vi "ASC-FlowControl.vi"() -> ()   [LabVIEW 2009]
uses:
  <vilib>/Utility/error.llb/DialogType.ctl
  Time_globals.vi
  Instance           4 19Saved   Wetlow_v1.2 .vi
panel:
  out "Flush":bool
  out "Progress":string
  in  "Fugacity table":dbl[](array[numeric])
  in  "Temperature table":dbl[](array[numeric])
  out "Fugacity":cluster{"Array":dbl[], "Array 2":dbl[]}[](graph)=[{"Array"=[17.44743958824043, 17.44743958824043], "Array 2"=[-15.0, -90.0]}, {"Array"=[14.85552997103172, 14.85552997103172], "Array 2"=[-15.0, -90.0]}, {"Array"=[12.93410075664489, 12.93410075664489], "Array 2"=[-15.0, -90.0]}, {"Array"=[11.45278589016778, 11.45278589016778], "Array 2"=[-15.0, -90.0]}, {"Array"=[10.27590813338129, 10.27590813338129], "Array 2"=[-15.0, -90.0]}, {"Array"=[9.318361831989936, 9.318361831989936], "Array 2"=[-15.0, -90.0]}, {"Array"=[21.13, 21.13], "Array 2"=[-15.0, -90.0]}, {"Array"=[26.8, 26.8], "Array 2"=[-15.0, -90.0]}, {"Array"=[33.65, 33.65], "Array 2"=[-15.0, -90.0]}, {"Array"=[9.0, 11.83374083129584, 33.65, 33.65], "Array 2"=[-17.9235, -25.63552567237164, -89.48, -89.48]}, {"Array"=[], "Array 2"=[]}] caption="XY Graph"
  in  "Continue":bool
  in  "Run Info Cluster In":T1
  out "Run Info Cluster Out":T1
  out "Datafile blob":string="8/29/2014\t3:28 PM\r\n\r\n0*C\r\nH2-CO2\r\nIW/IM+0\r\n\r\nTime\tSet_point\tLoad_end\tSample\tFan_end\tFan\tField\t%CO2\r\n"
  out "Stable":bool
  out "Off (*C)":dbl
  out "On (*C)":dbl
  out "Start":bool
  out "Cool":bool
  out "Time elapsed":bool
  in  "stop":bool
  out "Initial ramp":bool
  out "SP reached":bool
  out "Current SP":dbl=50.0
  out "Array":dbl[](array[numeric])
  out "refnum out":refnum<file>
  in  "Field":bool
  out "Field on":bool
  out "Fan on":bool
  in  "FAN":bool caption="Fan"
  in  "error in":errorcluster
  in  "Soak Time (min)":u32
  out "Field (uT)":dbl
  in  "Set Point (*C)":u32
  out "Time at Set Point":dbl format="%#.0f"
  out "Elapsed Time":dbl format="%#.0f"
  out "fan end":u32
  out "load end":u32
  out "sample":u32
  out "Watlow Chart":T2(graph)={"Number"=133, "Number"=270, "Number"=56}
  # "Temperature"
  # "Current\nTemperature"
  # "800"
  # "700"
  # "600"
  # "500"
  # "400"
  # "300"
  # "200"
  # "100"
  # "20"
  # "Temperature (*C)"
  # "User Information"
  # "Run Information"
  # "Run Information"
  # "User Information"
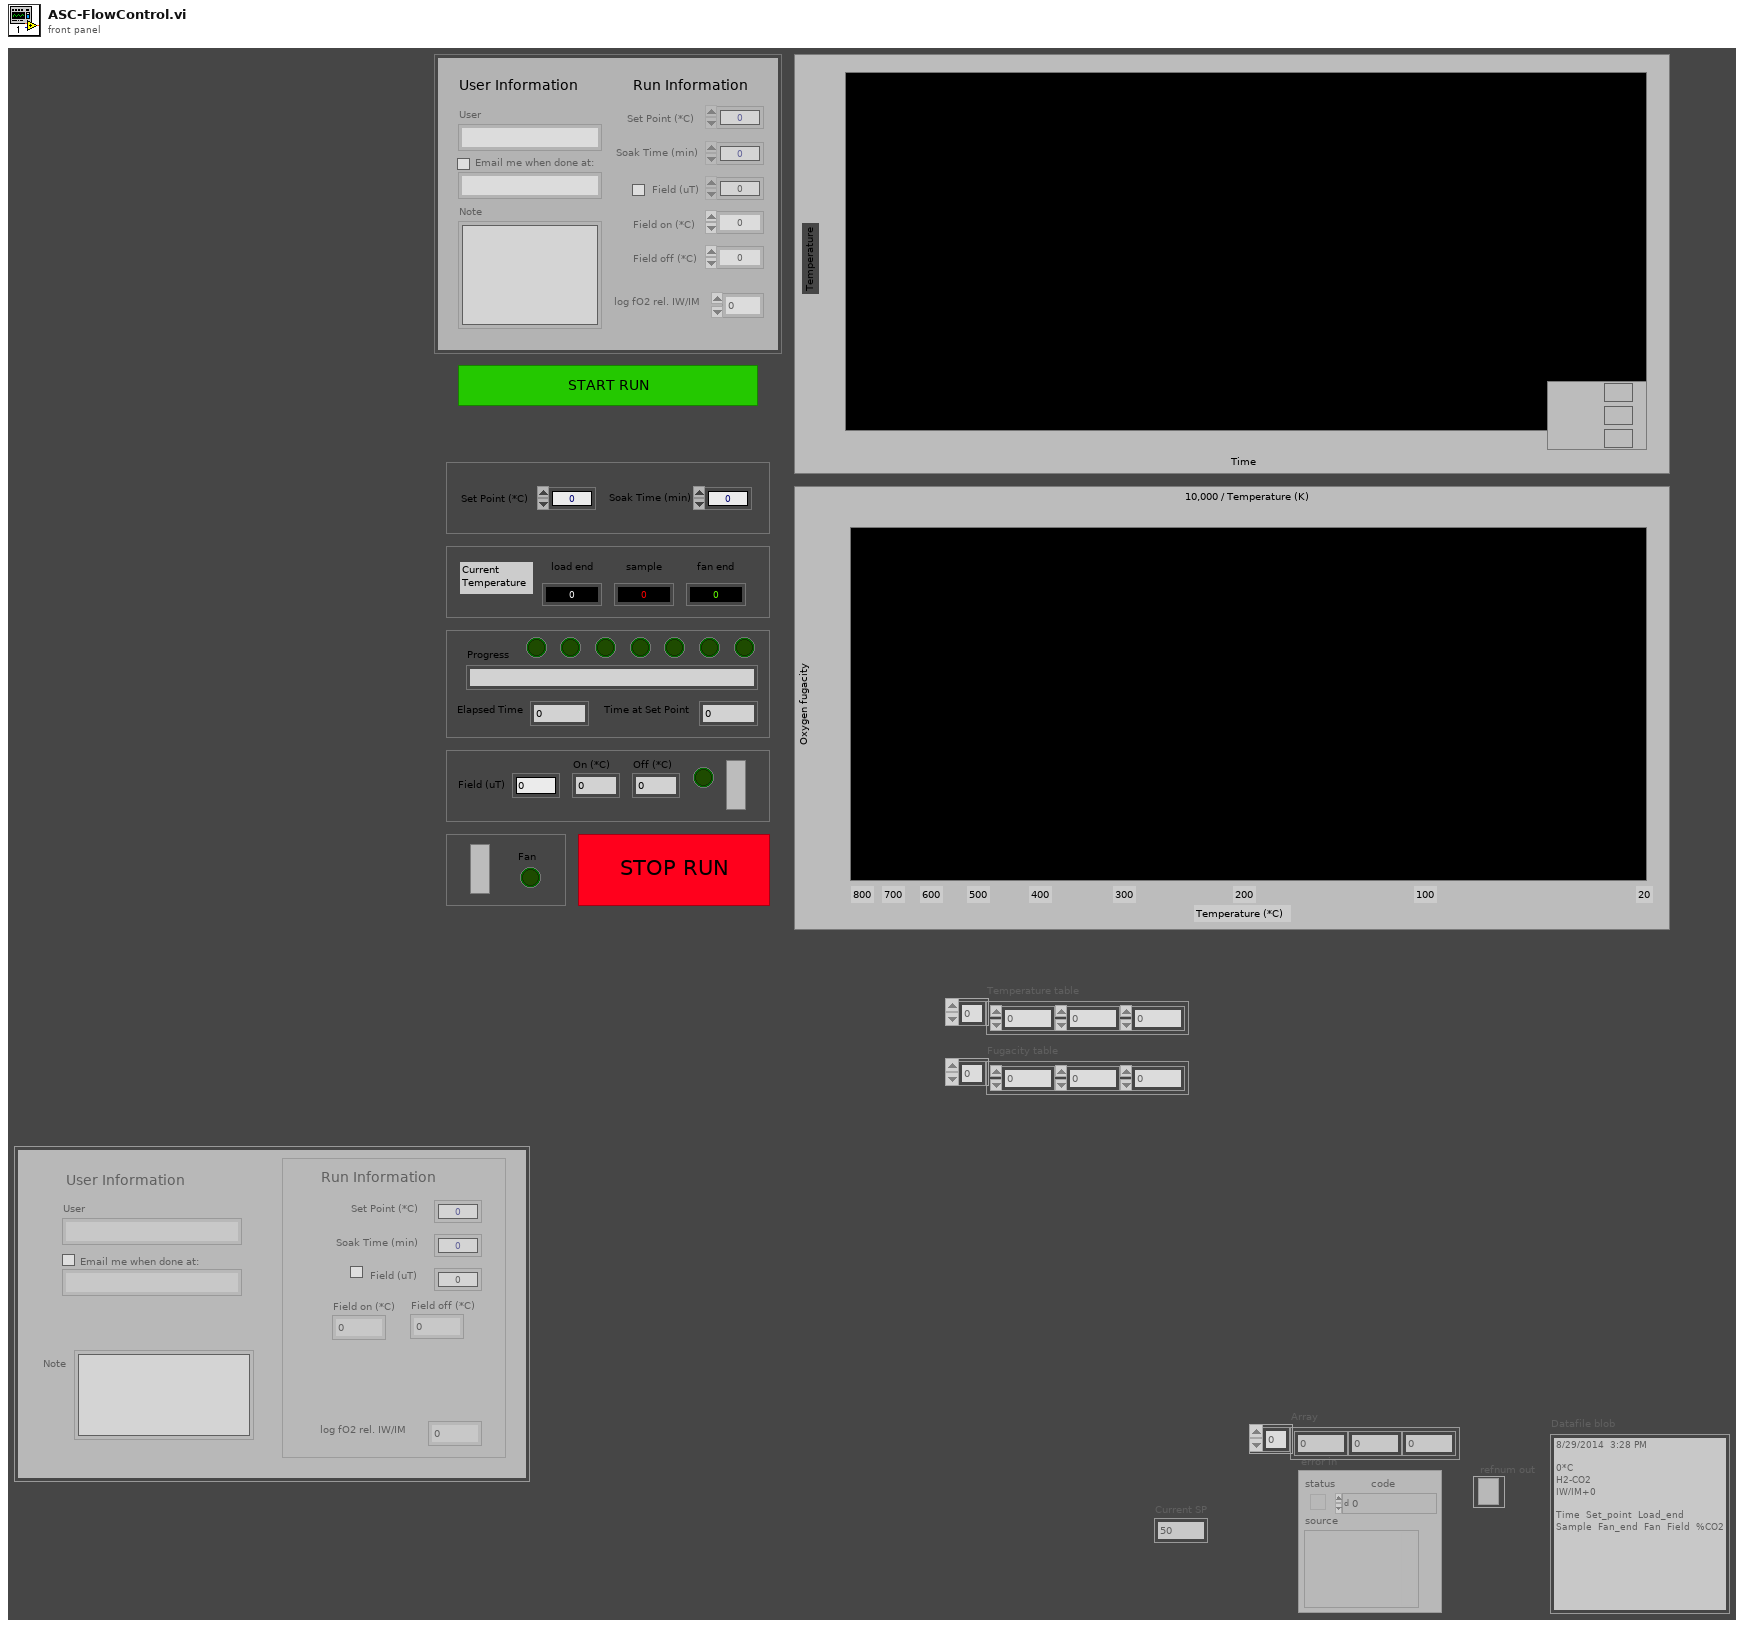
[diagram p1: front panel]
types:
  T1 = cluster{"Set Point (*C)":u32, "Field (uT)":dbl, "Soak Time (min)":u32, "User":string, "Note":string, "email address":string, "Email":bool, "Field on (*C)":dbl, "Field off (*C)":dbl, "Enable field":bool, "log fO2 rel. IW/IM":dbl}
  T2 = cluster{"Number":u32, "Number":u32, "Number":u32}
  T3 = cluster{"Number":u32, "Number":u32, "Number":u32}[]
  T4 = cluster{"Flow Controllers":refnum<visa-resource-name>, "Oven Fan":refnum<visa-resource-name>, "Oven Watlows":refnum<visa-resource-name>, "Field Power Supply":refnum<visa-resource-name>}
  T5 = typedef "DialogType.ctl" = u16
  T6 = cluster{"Oven Watlows":refnum<visa-resource-name>, "Field Power Supply":refnum<visa-resource-name>, "Oven Fan":refnum<visa-resource-name>, "Flow Controllers":refnum<visa-resource-name>}
  T7 = cluster{"Field on (*C)":dbl, "Field off (*C)":dbl, "Field (uT)":dbl, "Enable field":bool}
  T8 = cluster{"Set Point (*C)":u32, "Number":u32, string, "email address":string, "refnum out":refnum<file>, "Email":bool}
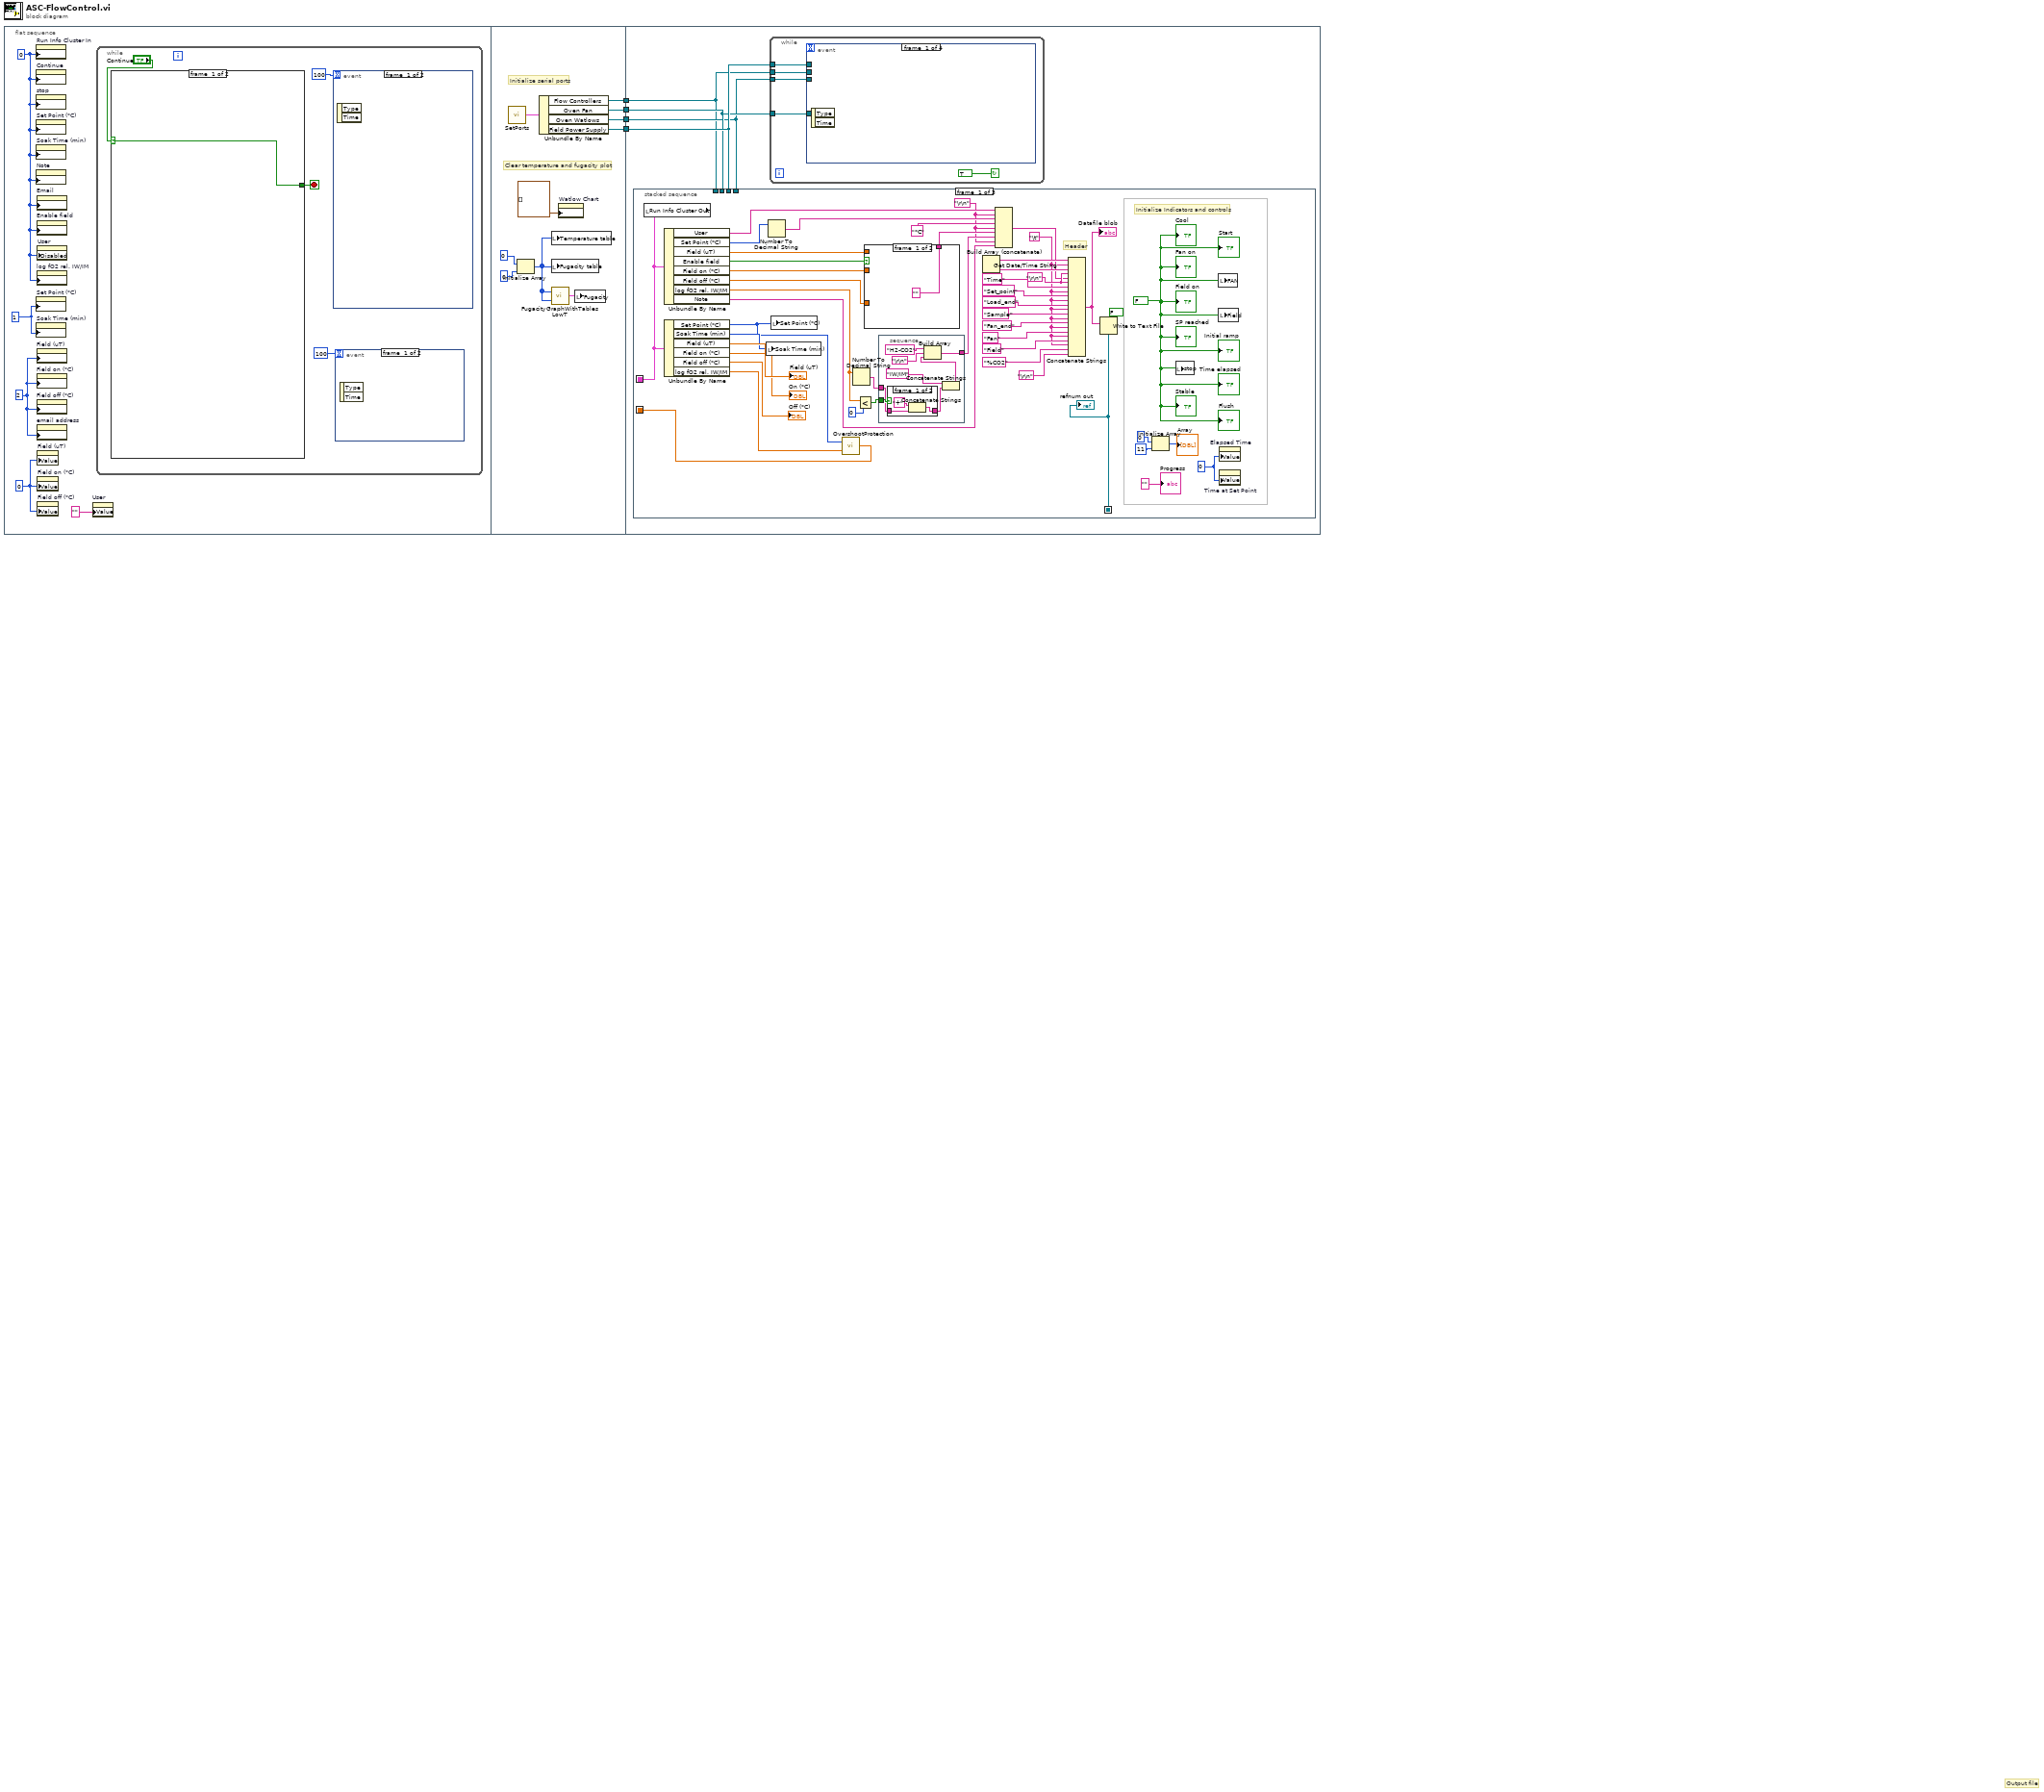
[diagram p0: block diagram]
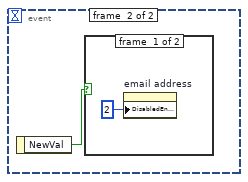
[diagram p2: hidden frame]
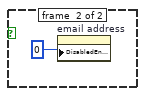
[diagram p3: hidden frame]
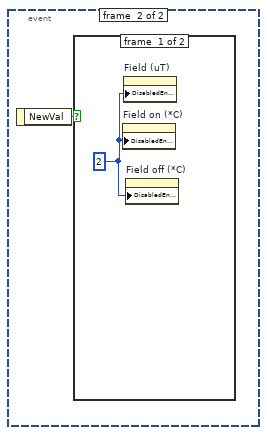
[diagram p4: hidden frame]
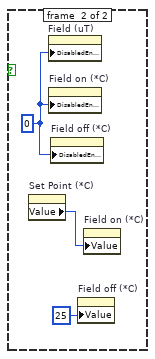
[diagram p5: hidden frame]
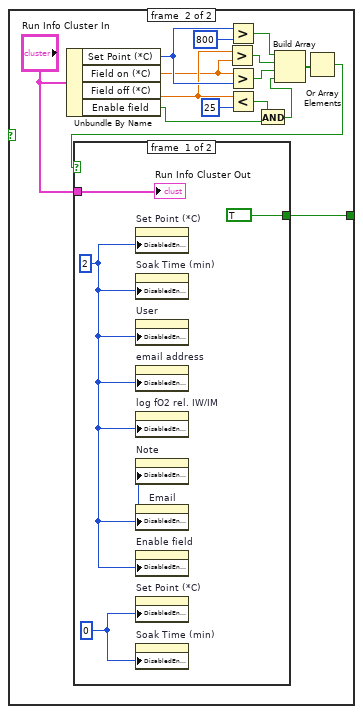
[diagram p6: hidden frame]
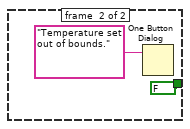
[diagram p7: hidden frame]
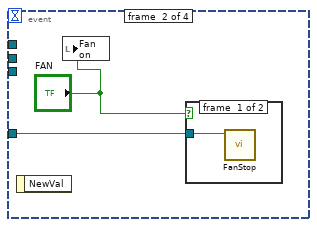
[diagram p8: hidden frame]
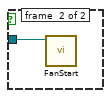
[diagram p9: hidden frame]
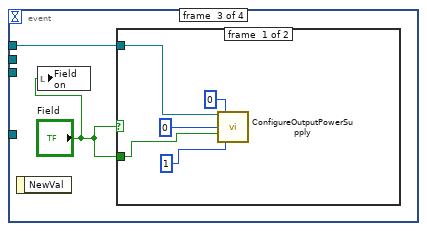
[diagram p10: hidden frame]
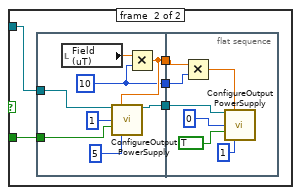
[diagram p11: hidden frame]
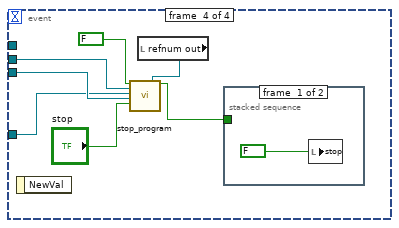
[diagram p12: hidden frame]
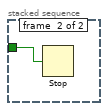
[diagram p13: hidden frame]
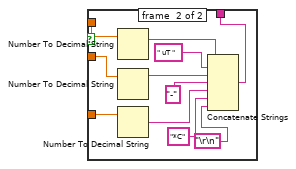
[diagram p15: hidden frame]
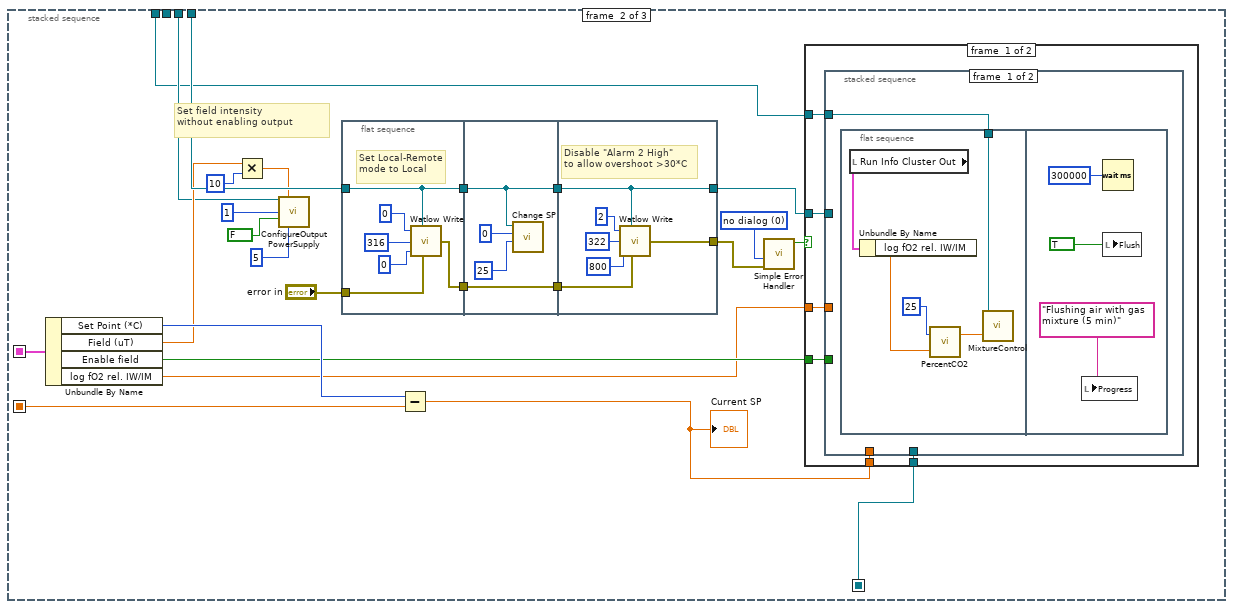
[diagram p16: hidden frame]
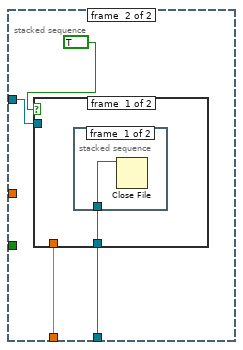
[diagram p17: hidden frame]
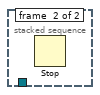
[diagram p18: hidden frame]
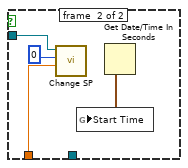
[diagram p19: hidden frame]
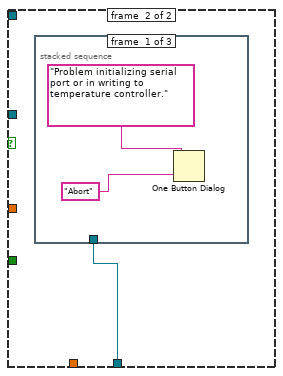
[diagram p20: hidden frame]
diagram:
  # "Output file"
  n1 = flat-sequence {
    tunnel: [w52] -> w4
    tunnel: [w51] -> w3
    tunnel: [w50] -> w2
    tunnel: [w47] -> w1
    tunnel: w4 -> [w57]
    tunnel: w3 -> [w56]
    tunnel: w2 -> [w55]
    tunnel: w1 -> [w54]
    frame #0 {
      w7 = 1
      w5 = 0
      w8 = 2
      w6 = 0
      n2 = property on="Run Info Cluster In" class="Clust (strict)"("DisabledEnum"=w5) -> ()  [unwired: 2 in, 2 out]
      n3 = property on="Continue" class="Bool (strict)"("DisabledEnum"=w5) -> ()  [unwired: 2 in, 2 out]
      n4 = property on="stop" class="Bool (strict)"("DisabledEnum"=w5) -> ()  [unwired: 2 in, 2 out]
      n5 = property on="Set Point (*C)" class="DigNum (strict)"("DisabledEnum"=w5) -> ()  [unwired: 2 in, 2 out]
      n6 = property on="Soak Time (min)" class="DigNum (strict)"("DisabledEnum"=w5) -> ()  [unwired: 2 in, 2 out]
      n7 = property on="Note" class="Str"("DisabledEnum"=w5) -> ()  [unwired: 2 in, 2 out]
      n8 = property on="Set Point (*C)" class="DigNum (strict)"("DisabledEnum"=w7) -> ()  [unwired: 2 in, 2 out]
      n9 = property on="Soak Time (min)" class="DigNum (strict)"("DisabledEnum"=w7) -> ()  [unwired: 2 in, 2 out]
      n10 = property on="Email" class="Bool (strict)"("DisabledEnum"=w5) -> ()  [unwired: 2 in, 2 out]
      n11 = property on="Enable field" class="Bool (strict)"("DisabledEnum"=w5) -> ()  [unwired: 2 in, 2 out]
      n12 = property on="log fO2 rel. IW/IM" class="DigNum (strict)"("DisabledEnum"=w5) -> ()  [unwired: 2 in, 2 out]
      n13 = property on="Field (uT)" class="DigNum (strict)"("DisabledEnum"=w8) -> ()  [unwired: 2 in, 2 out]
      n14 = property on="Field on (*C)" class="DigNum (strict)"("DisabledEnum"=w8) -> ()  [unwired: 2 in, 2 out]
      n15 = property on="Field off (*C)" class="DigNum (strict)"("DisabledEnum"=w8) -> ()  [unwired: 2 in, 2 out]
      n16 = property on="email address" class="Str"("DisabledEnum"=w8) -> ()  [unwired: 2 in, 2 out]
      n17 = property on="User" class="Str"("Disabled"=w5) -> ()  [unwired: 2 in, 2 out]
      n18 = property on="Field (uT)" class="DigNum (strict)"("Value"=w6) -> ()  [unwired: 2 in, 2 out]
      n19 = property on="Field on (*C)" class="DigNum (strict)"("Value"=w6) -> ()  [unwired: 2 in, 2 out]
      n20 = property on="Field off (*C)" class="DigNum (strict)"("Value"=w6) -> ()  [unwired: 2 in, 2 out]
      n21 = property on="User" class="Str"("Value"="") -> ()  [unwired: 2 in, 2 out]
      n22 = while {
        stop <- w12 stop-if-true
        n23 = case shown="True" "Continue" {
          selector: "Continue" -> [w22 _]
          tunnel: [w22 w36] -> w12
          frame #0 {
          }
          frame #1 {
            n24 = Unbundle By Name("Run Info Cluster In") -> ("Set Point (*C)"=w33:u32, "Field on (*C)"=w26:dbl, "Field off (*C)"=w27:dbl, "Enable field"=w24:bool)
            n25 = Greater?(x=w27, y=w26) -> (0:w28:bool)
            n26 = Greater?(x=w33, y=u32 800) -> (0:w32:bool)
            n27 = Greater?(x=w26, y=w33) -> (0:w31:bool)
            n28 = Less?(x=w27, y=25) -> (x < y?=w25:bool)
            n29 = And(x=w25, y=w24) -> (x .and. y?=w23:bool)
            n30 = Build Array(w32, w28, w31, w23) -> (w30:bool[])
            n31 = Or Array Elements(Boolean array=w30) -> (logical OR=w29:bool)
            n32 = case shown="False" w29 {
              tunnel: [TRUE FALSE] -> w36
              tunnel: "Run Info Cluster In" -> [w40 _]
              frame #0 {
                w38 = 0
                w39 = 2
                n33 = property on="Set Point (*C)" class="DigNum (strict)"("DisabledEnum"=w39) -> ()  [unwired: 2 in, 2 out]
                n34 = property on="Soak Time (min)" class="DigNum (strict)"("DisabledEnum"=w39) -> ()  [unwired: 2 in, 2 out]
                n35 = property on="User" class="Str"("DisabledEnum"=w39) -> ()  [unwired: 2 in, 2 out]
                n36 = property on="email address" class="Str"("DisabledEnum"=w39) -> ()  [unwired: 2 in, 2 out]
                n37 = property on="log fO2 rel. IW/IM" class="DigNum (strict)"("DisabledEnum"=w39) -> ()  [unwired: 2 in, 2 out]
                n38 = property on="Note" class="Str"("DisabledEnum"=w39) -> ()  [unwired: 2 in, 2 out]
                n39 = property on="Email" class="Bool (strict)"("DisabledEnum"=w39) -> ()  [unwired: 2 in, 2 out]
                n40 = property on="Enable field" class="Bool (strict)"("DisabledEnum"=w39) -> ()  [unwired: 2 in, 2 out]
                n41 = property on="Set Point (*C)" class="DigNum (strict)"("DisabledEnum"=w38) -> ()  [unwired: 2 in, 2 out]
                n42 = property on="Soak Time (min)" class="DigNum (strict)"("DisabledEnum"=w38) -> ()  [unwired: 2 in, 2 out]
                "Run Info Cluster Out" <- w40
              }
              frame #1 {
                n43 = One Button Dialog(message="Temperature set out of bounds.") -> ()  [unwired: 2 out]
              }
            }
          }
        }
        n44 = event shown="[1] \"Run Info Cluster In.Enable field\": Value Change" {
          selector: _ -> [_ _]
          dyn-events: _ -> [_ _]
          timeout: 100 -> [_ _]
          event #0 {
            n45 = event-data() -> ()  [unwired: 1 in, 2 out]
          }
          event #1 {
            n46 = event-data() -> ("NewVal"=w17:bool)  [unwired: 1 in]
            n47 = case shown="True" w17 {
              frame #0 {
                w18 = 2
                n48 = property on="Field on (*C)" class="DigNum (strict)"("DisabledEnum"=w18) -> ()  [unwired: 2 in, 2 out]
                n49 = property on="Field (uT)" class="DigNum (strict)"("DisabledEnum"=w18) -> ()  [unwired: 2 in, 2 out]
                n50 = property on="Field off (*C)" class="DigNum (strict)"("DisabledEnum"=w18) -> ()  [unwired: 2 in, 2 out]
              }
              frame #1 {
                w21 = 0
                n51 = property on="Set Point (*C)" class="DigNum (strict)"() -> ("Value"=w20:u32)  [unwired: 2 in, 2 out]
                n52 = property on="Field (uT)" class="DigNum (strict)"("DisabledEnum"=w21) -> ()  [unwired: 2 in, 2 out]
                n53 = property on="Field on (*C)" class="DigNum (strict)"("DisabledEnum"=w21) -> ()  [unwired: 2 in, 2 out]
                n54 = property on="Field off (*C)" class="DigNum (strict)"("DisabledEnum"=w21) -> ()  [unwired: 2 in, 2 out]
                n55 = property on="Field off (*C)" class="DigNum (strict)"("Value"=25) -> ()  [unwired: 2 in, 2 out]
                n56 = property on="Field on (*C)" class="DigNum (strict)"("Value"=w20) -> ()  [unwired: 2 in, 2 out]
              }
            }
          }
        }
        n57 = event shown="[1] \"Run Info Cluster In.Email\": Value Change" {
          selector: _ -> [_ _]
          dyn-events: _ -> [_ _]
          timeout: 100 -> [_ _]
          event #0 {
            n58 = event-data() -> ()  [unwired: 1 in, 2 out]
          }
          event #1 {
            n59 = event-data() -> ("NewVal"=w14:bool)  [unwired: 1 in]
            n60 = case shown="False" w14 {
              frame #0 {
                n61 = property on="email address" class="Str"("DisabledEnum"=2) -> ()  [unwired: 2 in, 2 out]
              }
              frame #1 {
                n62 = property on="email address" class="Str"("DisabledEnum"=0) -> ()  [unwired: 2 in, 2 out]
              }
            }
          }
        }
      }
    }
    frame #1 {
      # "Clear temperature and fugacity plot"
      # "Initialize serial ports"
      n63 = call "SetPorts.vi"() -> ("Ports"=w53:T4)  [unwired: 1 in]
      n64 = Initialize Array(0, 0) -> (w46:i32[])
      n65 = Unbundle By Name(w53) -> ("Flow Controllers"=w47:refnum<visa-resource-name>, "Oven Fan"=w51:refnum<visa-resource-name>, "Oven Watlows"=w50:refnum<visa-resource-name>, "Field Power Supply"=w52:refnum<visa-resource-name>)
      n66 = local write "Temperature table"(w46) -> ()
      n67 = local write "Fugacity table"(w46) -> ()
      n68 = call "FugacityGraphWithTablesLowT.vi"("Fugacity table"=w46, "Temperature table"=w46) -> ("Array"=w45:cluster{"Array":dbl[], "Array 2":dbl[]}[])
      n69 = property on="Watlow Chart" class="WaveformChart (strict)"("History Data"=T3 []) -> ()  [unwired: 2 in, 2 out]
      n70 = local write "Fugacity"(w45) -> ()
    }
    frame #2 {
      n71 = stacked-sequence {
        seq-local: [w106 _ _] -> [_ w174 w257]
        seq-local: [w111 _ _] -> [_ w195 w253]
        seq-local: [w103 _ _] -> [_ w191 _]
        tunnel: w55 -> [_ w192 w251]
        tunnel: w56 -> [_ _ w243]
        tunnel: w57 -> [_ w182 w255]
        tunnel: w54 -> [_ w173 w252]
        frame #0 {
          (unwired) FALSE ("SP reached")
          w118 = "\r\n" ("End of Line Constant")
          w136 = "\r\n" ("End of Line Constant")
          w110 = "\t" ("Tab Constant")
          w108 = FALSE
          w147 = 0
          # "Header"
          # "Initialize Indicators and controls"
          n72 = local read "Run Info Cluster Out"() -> (w111:T1)
          n73 = Unbundle By Name(w111) -> ("User"=w127:string, "Set Point (*C)"=w132:u32, "Field (uT)"=w122:dbl, "Enable field"=w123:bool, "Field on (*C)"=w120:dbl, "Field off (*C)"=w119:dbl, "log fO2 rel. IW/IM"=w114:dbl, "Note"=w117:string)
          n74 = Unbundle By Name(w111) -> ("Set Point (*C)"=w105:u32, "Soak Time (min)"=w141:u32, "Field (uT)"=→"Field (uT)":dbl, "Field on (*C)"=→"On (*C)":dbl, "Field off (*C)"=→"Off (*C)":dbl, "log fO2 rel. IW/IM"=w104:dbl)
          n75 = local write "Soak Time (min)"(w141) -> ()
          n76 = Number To Decimal String(number=w132) -> (decimal integer string=w131:string)  [unwired: 1 out]
          n77 = local write "Set Point (*C)"(w105) -> ()
          n78 = call "OvershootProtection.vi"("Log fO2 rel. IW/IM"=w104, "Set Point (*C)"=w105) -> ("Overshoot protection"=w103:dbl)
          n79 = Number To Decimal String(number=w114) -> (decimal integer string=w116:string)  [unwired: 1 out]
          n80 = Less?(x=w114, y=0) -> (x < y?=w113:bool)
          n81 = case shown="True" w123 {
            tunnel: w122 -> [_ w172]
            tunnel: ["" w163] -> w121
            tunnel: w120 -> [_ w169]
            tunnel: w119 -> [_ w168]
            frame #0 {
            }
            frame #1 {
              n82 = Number To Decimal String(number=w172) -> (decimal integer string=w171:string)  [unwired: 1 out]
              n83 = Number To Decimal String(number=w169) -> (decimal integer string=w167:string)  [unwired: 1 out]
              n84 = Number To Decimal String(number=w168) -> (decimal integer string=w166:string)  [unwired: 1 out]
              n85 = Concatenate Strings(w171, " uT ", w167, "-", w166, "*C", "\r\n" ("End of Line Constant")) -> (w163:string)
            }
          }
          n86 = stacked-sequence {
            tunnel: [w155] -> w129
            tunnel: w116 -> [w150]
            tunnel: w113 -> [w151]
            frame #0 {
              n87 = case shown="True" w151 {
                tunnel: w150 -> [w158 w160]
                tunnel: [w157 w160] -> w149
                frame #0 {
                  n88 = Concatenate Strings("+", w158) -> (w157:string)
                }
                frame #1 {
                }
              }
              n89 = Concatenate Strings("IW/IM", w149) -> (w152:string)
              n90 = Build Array("H2-CO2", "\r\n" ("End of Line Constant"), w152) -> (w155:string[])
            }
          }
          n91 = Get Date/Time String() -> (date string=w138:string, time string=w137:string)  [unwired: 3 out]
          n92 = Build Array (concatenate)(w127, w118, w131, "*C", w118, w121, w129, w118, w117) -> (w128:string[])
          n93 = Concatenate Strings(w138, w110, w137, w136, w128, w136, "Time", w110, "Set_point", w110, "Load_end", w110, "Sample", w110, "Fan_end", w110, "Fan", w110, "Field", w110, "%CO2", "\r\n") -> (w112:string)
          "Datafile blob" <- w112
          n94 = Write to Text File(text=w112) -> (refnum out=w106:refnum<file>)  [unwired: 1 in, 4 out]
          "refnum out" <- w106
          n95 = Initialize Array(0, 11) -> (→"Array":i32[])
          n96 = local write "stop"(w108) -> ()
          n97 = local write "FAN"(w108) -> ()
          n98 = local write "Field"(w108) -> ()
          n99 = property on="Elapsed Time" class="DigNum (strict)"("Value"=w147) -> ()  [unwired: 2 in, 2 out]
          n100 = property on="Time at Set Point" class="DigNum (strict)"("Value"=w147) -> ()  [unwired: 2 in, 2 out]
          "Fan on" <- w108
          "Field on" <- w108
          "SP reached" <- w108
          "Initial ramp" <- w108
          "Cool" <- w108
          "Stable" <- w108
          "Time elapsed" <- w108
          "Start" <- w108
          "Flush" <- w108
          "Progress" <- ""
        }
        frame #1 {
          w197 = T5 0 items=["no dialog", "OK message", "continue or stop message", "OK message + warnings", "continue/stop + warnings"] ("type of dialog (OK msg:1)")
          # "Set field intensity\nwithout enabling output"
          n101 = Unbundle By Name(w195) -> ("Set Point (*C)"=w194:u32, "Field (uT)"=w183:dbl, "Enable field"=w181:bool, "log fO2 rel. IW/IM"=w180:dbl)
          n102 = Multiply(x=w183, y=10) -> (x*y=w185:dbl)
          n103 = call "ConfigureOutputPowerSupply.vi"("VISA resource name"=w182, "Manual Range(0.00)"=w185, "Function(0:Voltage)"=1, "Output Enable (T: Enable)"=FALSE, "Unit(V)"=5) -> ()  [unwired: 9 in, 2 out]
          n104 = flat-sequence {
            tunnel: w192 -> [w200]
            tunnel: [w200] -> w179
            tunnel: "error in" -> [w199]
            tunnel: [w198] -> w177
            tunnel: w179 -> [w206]
            tunnel: [w206] -> w178
            tunnel: w177 -> [w207]
            tunnel: [w207] -> w176
            tunnel: w178 -> [w208]
            tunnel: w176 -> [w213]
            tunnel: [w209] -> w175
            tunnel: [w208] -> w190
            frame #0 {
              # "Set Local-Remote\nmode to Local"
              n105 = call "Watlow Write.vi"("Adress"=0, "VISA resource name"=w200, "Register"=316, "Parameter"=0, "error in (no error)"=w199) -> ("error out"=w198:errorcluster)
            }
            frame #1 {
              n106 = call "Change SP.vi"("Set Point"=25, "Adress"=0, "VISA resource name"=w206) -> ()  [unwired: 1 in, 1 out]
            }
            frame #2 {
              # "Disable \"Alarm 2 High\"\nto allow overshoot >30*C"
              n107 = call "Watlow Write.vi"("Adress"=2, "VISA resource name"=w208, "Register"=322, "Parameter"=800, "error in (no error)"=w213) -> ("error out"=w209:errorcluster)
            }
          }
          n108 = Subtract(x=w194, y=w191) -> (x-y=w189:dbl)
          "Current SP" <- w189
          n109 = call <vilib>:"Simple Error Handler.vi"("type of dialog (OK msg:1)"=w197, "error in (no error)"=w175) -> ("error?"=w196:bool)  [unwired: 7 out]
          n110 = case shown="False" w196 {
            tunnel: w174 -> [w219 w239]
            tunnel: w190 -> [w218 _]
            tunnel: w189 -> [w217 _]
            tunnel: w181 -> [w216 _]
            tunnel: w180 -> [w215 _]
            tunnel: w173 -> [w214 _]
            frame #0 {
              n111 = stacked-sequence {
                tunnel: w219 -> [_ w232]
                tunnel: w218 -> [_ w231]
                tunnel: w217 -> [_ w230]
                tunnel: w216 -> [_ _]
                tunnel: w215 -> [_ _]
                tunnel: w214 -> [w220 _]
                frame #0 {
                  n112 = flat-sequence {
                    tunnel: w220 -> [w225]
                    frame #0 {
                      n113 = local read "Run Info Cluster Out"() -> (w224:T1)
                      n114 = Unbundle By Name(w224) -> ("log fO2 rel. IW/IM"=w223:dbl)
                      n115 = call "PercentCO2.vi"("log fO2 rel. IW/IM"=w223, "Temperature"=25) -> ("%CO2"=w222:dbl)  [unwired: 1 out]
                      n116 = call "MixtureControl.vi"("%CO2"=w222, "VISA resource name"=w225) -> ()  [unwired: 1 in]
                    }
                    frame #1 {
                      n117 = local write "Progress"("Flushing air with gas mixture (5 min)") -> ()
                      n118 = Wait (ms)(milliseconds to wait=300000) -> ()  [unwired: 1 out]
                      n119 = local write "Flush"(TRUE) -> ()
                    }
                  }
                }
                frame #1 {
                  n120 = case shown="True" TRUE {
                    tunnel: w232 -> [w233 _]
                    tunnel: w231 -> [_ w237]
                    tunnel: w230 -> [_ w236]
                    frame #0 {
                      n121 = stacked-sequence {
                        tunnel: w233 -> [w234 _]
                        frame #0 {
                          n122 = Close File(refnum=w234) -> ()  [unwired: 1 in, 2 out]
                        }
                        frame #1 {
                          n123 = Stop() -> ()  [unwired: 1 out]
                        }
                      }
                    }
                    frame #1 {
                      n124 = call "Change SP.vi"("Set Point"=w236, "Adress"=0, "VISA resource name"=w237) -> ()  [unwired: 1 in, 1 out]
                      n125 = Get Date/Time In Seconds() -> (seconds since 1Jan1904=w238:timestamp)
                      n126 = global write "Time_globals.vi" "Start Time"(w238) -> ()
                    }
                  }
                }
              }
            }
            frame #1 {
              n127 = stacked-sequence {
                tunnel: w239 -> [_ w242 _]
                frame #0 {
                  n128 = One Button Dialog(message="Problem initializing serial port or in writing to temperature controller.", button name ("OK")="Abort") -> ()  [unwired: 1 out]
                }
                frame #1 {
                  n129 = Close File(refnum=w242) -> ()  [unwired: 1 in, 2 out]
                }
                frame #2 {
                  n130 = Stop() -> ()  [unwired: 1 out]
                }
              }
            }
          }
        }
        frame #2 {
          n131 = Unbundle By Name(w253) -> ("log fO2 rel. IW/IM"=w244:dbl, "Field on (*C)"=w245:dbl, "Field off (*C)"=w246:dbl, "Field (uT)"=w247:dbl, "Enable field"=w248:bool, "email address"=w250:string, "Email"=w249:bool)
          n132 = local write "Progress"("Initial heating") -> ()
          n133 = local write "Start"(TRUE) -> ()
          n134 = call "FanStop.vi"("VISA resource name"=w243) -> ()  [unwired: 11 in]
          n135 = while {
            tunnel: w257 -> [w311]
            tunnel: w247 -> [w277]
            tunnel: w245 -> [w279]
            tunnel: w246 -> [w278]
            tunnel: w248 -> [w276]
            tunnel: w251 -> [w287]
            tunnel: w255 -> [w272]
            tunnel: w243 -> [w271]
            tunnel: w244 -> [w302]
            tunnel: w252 -> [w270]
            tunnel: w249 -> [w286]
            tunnel: w250 -> [w285]
            tunnel: w252 -> [w274]
            tunnel: w251 -> [w273]
            tunnel: w251 -> [w267]
            stop <- w284 stop-if-true
            w292 = "\t"
            # "Store sample temperature in array"
            # "Write data to file"
            # "Progress of sequence: change set point, control fan and field during cooling"
            # "Adjust gas mixture"
            # "Plot fugacity"
            # "Store sample inverse temperature in table"
            # "Plot temperatures"
            # "Read temperatures"
            n136 = global read "Time_globals.vi" "Start Time"() -> (w323:timestamp)
            n137 = local read "Array"() -> (w282:dbl[])
            n138 = Get Date/Time In Seconds() -> (seconds since 1Jan1904=w322:timestamp)
            n139 = for {
              N: 3 -> [_]
              tunnel: [w385] -> w331 mode=indexing
              tunnel: w287 -> [w384]
              i -> [w387]
              n140 = Increment(x=w387) -> (x+1=w386:i32)
              n141 = call "Watlow Read.vi"("Adress"=w386, "Register"=u8 100 ("ST-H"), "VISA resource name"=w384) -> ("Number"=w385:u32)  [unwired: 1 in, 2 out]
            }
            n142 = Bundle("Oven Watlows"=w273, "Field Power Supply"=w272, "Oven Fan"=w271, "Flow Controllers"=w270) -> (w269:T6)  [unwired: 1 in]
            n143 = Bundle("Field on (*C)"=w279, "Field off (*C)"=w278, "Field (uT)"=w277, "Enable field"=w276) -> (w275:T7)  [unwired: 1 in]
            n144 = Wait (ms)(milliseconds to wait=u32 5000) -> ()  [unwired: 1 out]
            n145 = Subtract(x=w322, y=w323) -> (x-y=w324:dbl)
            n146 = Divide(x=w324, y=60.0) -> (x/y=w259:dbl)
            "Elapsed Time" <- w259
            n147 = local read "Current SP"() -> (w280:dbl)
            n148 = Index Array(array=w331, index=0) -> (element=w327:u32)
            "load end" <- w327
            n149 = Index Array(array=w331, index=1) -> (element=w261:u32)
            "sample" <- w261
            n150 = Insert Into Array(array=w282, index=0, new element=w261) -> (w283:dbl[])
            n151 = Index Array(array=w331, index=2) -> (element=w326:u32)
            "fan end" <- w326
            n152 = local read "Time elapsed"() -> (w268:bool)
            n153 = local read "SP reached"() -> (w258:bool)
            n154 = Multiply(x=u32 60, y="Soak Time (min)") -> (x*y=w316:u32)
            n155 = Not(x=w258) -> (.not. x?=w266:bool)
            n156 = call "Elapsed Time2"("Time Target (s)"=w316, "Reset"=w266) -> ("Elapsed Time (s)"=w310:dbl, "Time has Elapsed"=w291:bool)  [unwired: 3 in, 13 out]
            n157 = Number To Decimal String(number=w327) -> (decimal integer string=w336:string)  [unwired: 1 out]
            n158 = Bundle("Number"=w327, "Number"=w261, "Number"=w326) -> (→"Watlow Chart":T2)  [unwired: 1 out]
            n159 = Number To Decimal String(number=w261) -> (decimal integer string=w330:string)  [unwired: 1 out]
            n160 = Less Or Equal?(x=w261, y=50) -> (x <= y?=w290:bool)
            n161 = Divide(x=w310, y=60.0) -> (x/y=→"Time at Set Point":dbl)
            n162 = local write "Time elapsed"(w291) -> ()
            n163 = Number To Decimal String(number=w326) -> (decimal integer string=w329:string)  [unwired: 1 out]
            n164 = And(x=w268, y=w290) -> (x .and. y?=w288:bool)
            n165 = case shown="False" w288 {
              tunnel: w302 -> [w341 w344]
              tunnel: w261 -> [w340 w345]
              tunnel: [w339 w342] -> w295
              tunnel: [w338 w343] -> w281
              tunnel: w274 -> [w337 _]
              frame #0 {
                n166 = call "PercentCO2.vi"("log fO2 rel. IW/IM"=w341, "Temperature"=w340) -> ("Fugacity"=w339:dbl, "%CO2"=w338:dbl)
                n167 = call "MixtureControl.vi"("%CO2"=w338, "VISA resource name"=w337) -> ()  [unwired: 1 in]
              }
              frame #1 {
                n168 = call "PercentCO2.vi"("log fO2 rel. IW/IM"=w344, "Temperature"=w345) -> ("Fugacity"=w342:dbl, "%CO2"=w343:dbl)
              }
            }
            n169 = Add(x=273.15, y=w261) -> (x+y=w299:dbl)
            n170 = local read "Field on"() -> (w307:bool)
            n171 = local read "Fan on"() -> (w308:bool)
            n172 = Number To Fractional String(number=w259, precision (6)=i16 1) -> (F-format string=w264:string)  [unwired: 2 out]
            n173 = case shown="True" w308 {
              tunnel: ["off" "on"] -> w313
              frame #0 {
              }
              frame #1 {
              }
            }
            n174 = Divide(x=10000, y=w299) -> (x/y=w297:dbl)
            n175 = case shown="False" w307 {
              tunnel: ["off" "on"] -> w314
              frame #0 {
              }
              frame #1 {
              }
            }
            n176 = Number To Decimal String(number=w280) -> (decimal integer string=w315:string)  [unwired: 1 out]
            n177 = Number To Fractional String(number=w281, precision (6)=2) -> (F-format string=w262:string)  [unwired: 2 in]
            n178 = Insert Into Array(array="Temperature table", new element=w297) -> (w296:dbl[])  [unwired: 1 in]
            n179 = Insert Into Array(array="Fugacity table", new element=w295) -> (w294:dbl[])  [unwired: 1 in]
            n180 = local read "Datafile blob"() -> (w305:string)
            n181 = local write "Fugacity table"(w294) -> ()
            n182 = Concatenate Strings(w264, w292, w315, w292, w336, w292, w330, w292, w329, w292, w313, w292, w314, w292, w262, "\r\n") -> (w318:string)
            n183 = Write to Text File(file (use dialog)=w311, text=w318) -> ()  [unwired: 1 in, 4 out]
            n184 = local write "Temperature table"(w296) -> ()
            n185 = call "FugacityGraphWithTablesLowT.vi"("Fugacity table"=w294, "Temperature table"=w296) -> ("Array"=→"Fugacity":cluster{"Array":dbl[], "Array 2":dbl[]}[])
            n186 = Concatenate Strings(w305, w318) -> (w304:string)
            n187 = case shown="False" w291 {
              tunnel: w311 -> [_ w368]
              tunnel: w304 -> [_ w379]
              tunnel: [FALSE w377] -> w284
              tunnel: "Set Point (*C)" -> [w359 w381]
              tunnel: w261 -> [w358 w380]
              tunnel: w267 -> [w357 _]
              tunnel: w286 -> [_ w370]
              tunnel: w285 -> [_ w369]
              tunnel: w283 -> [w361 _]
              tunnel: w280 -> [w360 _]
              tunnel: w275 -> [_ w367]
              tunnel: w269 -> [_ w366]
              tunnel: w259 -> [w350 _]
              frame #0 {
                n188 = local read "Initial ramp"() -> (w363:bool)
                n189 = local read "Stable"() -> (w364:bool)
                n190 = local read "SP reached"() -> (w365:bool)
                n191 = call "ProgressControl.vi"("Elapsed time IN"=w350, "SP IN"=w359, "Array IN"=w361, "Current SP IN"=w360, "Stable"=w364, "Initial ramp IN"=w363, "SP reached IN"=w365, "Oven Watlows"=w357, "Sample"=w358) -> ("Array"=w362:dbl[], "Progress"=w356:string, "Current SP"=w355:dbl, "Stable"=w354:bool, "Initial ramp"=w353:bool, "SP reached"=w351:bool)  [unwired: 5 in]
                n192 = local write "SP reached"(w351) -> ()
                n193 = local write "Array"(w362) -> ()
                n194 = local write "Initial ramp"(w353) -> ()
                n195 = local write "Stable"(w354) -> ()
                n196 = local write "Current SP"(w355) -> ()
                n197 = local write "Progress"(w356) -> ()
              }
              frame #1 {
                n198 = Bundle("Set Point (*C)"=w381, "Number"=w380, w379, "email address"=w369, "refnum out"=w368, "Email"=w370) -> (w378:T8)  [unwired: 1 in]
                n199 = local read "Fan on"() -> (w376:bool)
                n200 = local read "Field on"() -> (w375:bool)
                n201 = call "Cooling.vi"("Read Field"=w375, "Read Fan"=w376, "Field"=w367, "Cluster"=w378, "Ports"=w366) -> ("Fan on"=w373:bool, "stop"=w371:bool, "Field on"=w374:bool, "Cool"=w377:bool, "Current SP"=w372:dbl)  [unwired: 2 in]
                n202 = local write "Current SP"(w372) -> ()
                n203 = local write "stop"(w371) -> ()
                n204 = local write "Field on"(w374) -> ()
                n205 = local write "Fan on"(w373) -> ()
                n206 = local write "Progress"("Cooling") -> ()
              }
            }
            n207 = local write "Cool"(w284) -> ()
            n208 = local write "Datafile blob"(w304) -> ()
          }
        }
      }
      n209 = while {
        tunnel: w55 -> [w61]
        tunnel: w56 -> [w60]
        tunnel: w57 -> [w59]
        tunnel: w54 -> [w58]
        stop <- TRUE continue-if-true
        n210 = event shown="[3] \"stop\": Value Change" {
          selector: _ -> [_ _ _ _]
          dyn-events: _ -> [_ _ _ _]
          timeout: _ -> [_ _ _ _]
          tunnel: w61 -> [_ _ _ w97]
          tunnel: w60 -> [_ w63 _ w96]
          tunnel: w59 -> [_ _ w67 _]
          tunnel: w58 -> [_ _ _ w95]
          event #0 {
            n211 = event-data() -> ()  [unwired: 1 in, 2 out]
          }
          event #1 {
            n212 = event-data() -> ()  [unwired: 1 in, 1 out]
            n213 = local write "Fan on"("FAN") -> ()
            n214 = case shown="True" "FAN" {
              tunnel: w63 -> [w65 w66]
              frame #0 {
                n215 = call "FanStop.vi"("VISA resource name"=w65) -> ()  [unwired: 11 in]
              }
              frame #1 {
                n216 = call "FanStart.vi"("VISA resource name"=w66) -> ()  [unwired: 11 in]
              }
            }
          }
          event #2 {
            n217 = event-data() -> ()  [unwired: 1 in, 1 out]
            n218 = local write "Field on"("Field") -> ()
            n219 = case shown="True" "Field" {
              tunnel: w67 -> [w70 w77]
              tunnel: "Field" -> [w69 w78]
              frame #0 {
                n220 = call "ConfigureOutputPowerSupply.vi"("VISA resource name"=w70, "Manual Range(0.00)"=0, "Function(0:Voltage)"=0, "Output Enable (T: Enable)"=w69, "Unit(V)"=1) -> ()  [unwired: 9 in, 2 out]
              }
              frame #1 {
                n221 = flat-sequence {
                  tunnel: w77 -> [w83]
                  tunnel: w78 -> [w82]
                  tunnel: [w81] -> w76
                  tunnel: [w80] -> w75
                  tunnel: [w79] -> w74
                  tunnel: w76 -> [w90]
                  tunnel: w75 -> [w89]
                  tunnel: w74 -> [w88]
                  frame #0 {
                    w79 = 10
                    n222 = local read "Field (uT)"() -> (w86:dbl)
                    n223 = Multiply(x=w86, y=w79) -> (x*y=w80:dbl)
                    n224 = call "ConfigureOutputPowerSupply.vi"("VISA resource name"=w83, "Manual Range(0.00)"=w80, "Function(0:Voltage)"=1, "Output Enable (T: Enable)"=w82, "Unit(V)"=5) -> ("VISA resource name out"=w81:refnum<visa-resource-name>)  [unwired: 9 in, 1 out]
                  }
                  frame #1 {
                    n225 = Multiply(x=w89, y=w88) -> (x*y=w87:dbl)
                    n226 = call "ConfigureOutputPowerSupply.vi"("VISA resource name"=w90, "Manual Range(0.00)"=w87, "Function(0:Voltage)"=0, "Output Enable (T: Enable)"=TRUE, "Unit(V)"=1) -> ()  [unwired: 9 in, 2 out]
                  }
                }
              }
            }
          }
          event #3 {
            n227 = event-data() -> ()  [unwired: 1 in, 1 out]
            n228 = local read "refnum out"() -> (w94:refnum<file>)
            n229 = call "stop_program.vi"("Run complete"=FALSE, "Flow Controllers"=w95, "Fan"=w96, "Watlows"=w97, "stop"="stop", "filename"=w94) -> ("Reset?"=w100:bool)  [unwired: 12 in, 1 out]
            n230 = stacked-sequence {
              tunnel: w100 -> [_ w102]
              frame #0 {
                n231 = local write "stop"(FALSE) -> ()
              }
              frame #1 {
                n232 = Stop(stop? (T)=w102) -> ()
              }
            }
          }
        }
      }
    }
  }
